vi "AssertVIExecState_Tests.vi"(11 "error in":errorcluster) -> (15 "error out":errorcluster)   [LabVIEW 2016, in "DronaTest.lvlib"]
uses:
  DronaTest.lvlib
  APIs/Assert/AssertVI/AssertVIExecNotBad.vi
  APIs/Assert/AssertVI/AssertVIExecRunning.vi
  APIs/Stimulus/VI/CloseVI.vi
  APIs/Assert/AssertVI/AssertVIExecIdle.vi
  <vilib>/addons/_JKI Toolkits/Caraya/classes/Assert/Assert True.vi
  <vilib>/addons/_JKI Toolkits/Caraya/classes/Test/Test.lvclass
  Drona.lvlib
  <vilib>/addons/_JKI Toolkits/Caraya/classes/Assert/Assert.lvclass
  APIs/Assert/AssertVI/AssertVI.lvlib
  APIs/Stimulus/VI/VI.lvlib
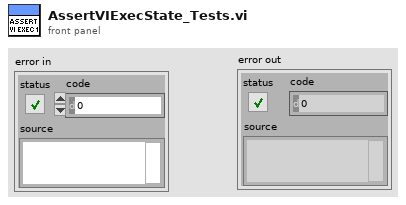
[diagram p1: front panel]
types:
  T1 = enum32{"Bad", "Idle", "Run top level", "Running"}[]
  T2 = enum32{"Bad", "Idle", "Run top level", "Running"}
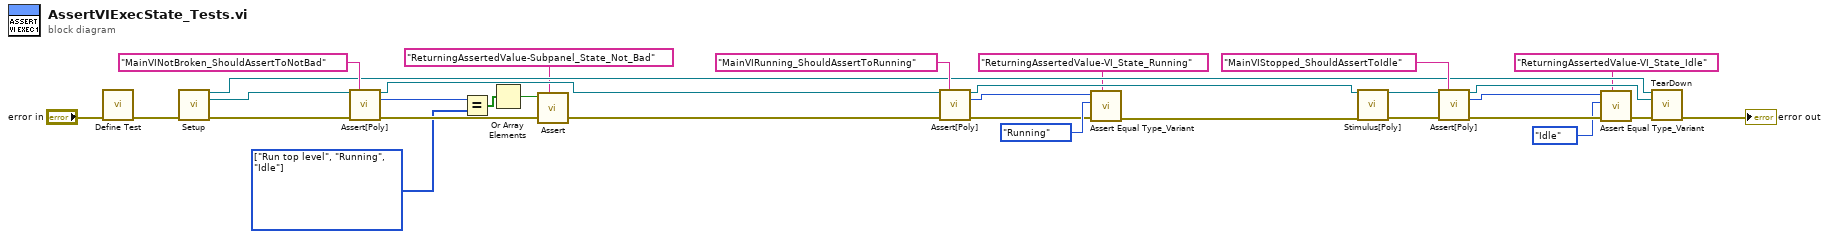
[diagram p0: block diagram]
diagram:
  w3 = T1 [enum."Run top level", enum."Running", enum."Idle"] items=["Bad", "Idle", "Run top level", "Running"] ("Execution:State")
  n1 = call <vilib>:"Define Test.vi"("error in (no error)"="error in") -> ("error out"=w26:errorcluster)  [unwired: 9 in, 1 out]
  n2 = call "Setup.vi"("error in (no error)"=w26) -> ("Application Ref"=w15:refnum<vi>, "VI out"=w19:refnum<vi>, "error out"=w20:errorcluster)  [unwired: 12 in]
  n3 = call-poly "Assert[Poly].vi"("VI Reference In"=w19, "Test Label"="MainVINotBroken_ShouldAssertToNotBad" ("Label"), "Error In"=w20) -> ("VI Reference Out"=w17:refnum<vi>, "Asserted Value"=w1:T2, "Error Out"=w18:errorcluster)  [unwired: 10 in]
  n4 = Equal?(x=w1, y=w3) -> (x = y?=w4:bool[])
  n5 = Or Array Elements(Boolean array=w4) -> (logical OR=w5:bool)
  n6 = call-poly <vilib>:"Assert.vi"("Label"="ReturningAssertedValue-Subpanel_State_Not_Bad", "True?"=w5) -> ()  [unwired: 8 in, 2 out]
  n7 = call-poly "Assert[Poly].vi"("VI Reference In"=w17, "Test Label"="MainVIRunning_ShouldAssertToRunning" ("Label"), "Error In"=w18) -> ("VI Reference Out"=w16:refnum<vi>, "Asserted Value"=w7:T2, "Error Out"=w9:errorcluster)  [unwired: 10 in]
  n8 = call <vilib>:"Assert Equal Type_Variant.vi"("Label"="ReturningAssertedValue-VI_State_Running", "error in (no error)"=w9, "Y"=T2."Running" ("Asserted Value"), "X"=w7) -> ("error out"=w8:errorcluster)  [unwired: 6 in, 1 out]
  n9 = call-poly "Stimulus[Poly].vi"("VI Reference In"=w16, "error in"=w8) -> ("VI Reference Out"=w24:refnum<vi>, "error out"=w25:errorcluster)  [unwired: 12 in]
  n10 = call-poly "Assert[Poly].vi"("VI Reference In"=w24, "Test Label"="MainVIStopped_ShouldAssertToIdle" ("Label"), "Error In"=w25) -> ("VI Reference Out"=w21:refnum<vi>, "Asserted Value"=w11:T2, "Error Out"=w22:errorcluster)  [unwired: 10 in]
  n11 = call <vilib>:"Assert Equal Type_Variant.vi"("Label"="ReturningAssertedValue-VI_State_Idle", "Y"=T2."Idle" ("Asserted Value"), "X"=w11) -> ()  [unwired: 7 in, 2 out]
  n12 = call "TearDown.vi"("Application Ref"=w15, "VI in"=w21, "error in (no error)"=w22) -> ("error out"=→"error out":errorcluster)  [unwired: 12 in]
